vi "Acq Configure Pretrigger Period.vi"(0 "session in":refnum<class "Digitizer Control.lvclass">, 1 "desired pre-trigger period (s)":dbl, 2 "TClk period (s)":dbl, 5 "error in (no error)":errorcluster) -> (14 "session out":refnum<class "Digitizer Control.lvclass">, 15 "actual pre-trigger period (s)":dbl, 16 "configured pre-trigger period (s)":dbl, 17 "additional samples to acquire (samples)":i64, 19 "error out":errorcluster)   [LabVIEW 2021, in "Digitizer Control.lvclass"]
doc: "Configures the acquisition pre-trigger period.\n\nInputs:\n\n<B>session in</B>: The device session.\n\n<B>desired pre-trigger period (s)</B>: The desired pre-trigger period, in seconds, to acquire before recognizing the start trigger. The actual pre-trigger period is returned on the <B>actual pre-trigger period (s)</B> output.\n\n<B>TClk period (s)</B>: The TClk clock period in seconds. TClk synchronized acquisitions have an inherent trigger response latency that is between 1-2 TClk periods. The latency can be compensated by acquiring additional pre-trigger samples and keeping only latency worth of the additional pre-trigger samples. Set this input to the TClk period to compensate for the trigger latency (following the <B>niTClk Synchronize.vi</B> call, read the Actual TClk:Period propery of a tclk session passed to the <B>niTClk Synchronize.vi</B> using a Property Node and pass the returned value on this input), this will increase the pre-trigger period configured on the FPGA Target by 2*<B>TClk period (s)</B>. The FPGA Target can record the actual trigger response latency for each trigger by enabling the trigger delay tracking (using the <B>trigger delay tracking enable</B> input of the <B>Acq Configure Transfer.vi</B>). The recorded latency values can be fetched by the <B>Acq Fetch Trigger Delay.vi</B>, which also returns the number of samples to remove from the beginning of the acquired waveform to keep only <B>actual pre-trigger period (s)</B> worth of pre-trigger samples.\n\nOutputs:\n\n<B>session out</B>: The device session passed on the <B>session in</B> input.\n\n<B>actual pre-trigger period (s)</B>: The actual pre-trigger period, in seconds.\n\n<B>configured pre-trigger period (s)</B>: The pre-trigger period configured on the FPGA Target, given in seconds, including the additional pre-trigger period for the TClk trigger response latency compensation (this output equals to <B>actual pre-trigger period (s)</B> + 2 * <B>TClk period (s)</B>).\n\n<B>additional samples to acquire (samples)</B>: The number of additional samples to acquire for the TClk trigger response latency compensation. This output is valid only if the <B>Acq Configure Channel.vi</B> has been already called on the session, otherwise this output returns zero."
uses:
  Digitizer Control.lvclass
  Digitizer Control.lvclass/Digitizer Control.ctl
  <vilib>/Utility/error.llb/Error Cluster From Error Code.vi
  <vilib>/rvi/errors/niLvFpgaAdjustHostInterfaceError.vi
  <vilib>/rvi/interface/nirviReadWriteControl/nirviReadWriteControl.xnode
  <vilib>/ErrorRing/Error Ring.xnode
  NiFpgaLv.dll
  <vilib>/rvi/interface/Simulation/niFpgaSimulationCallBeginRW.vi
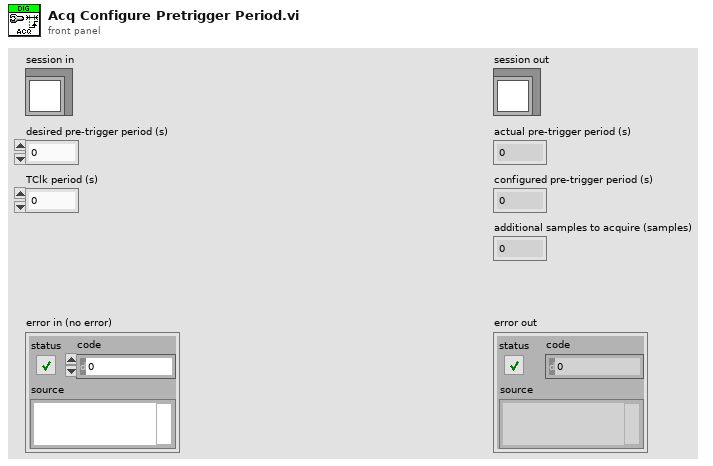
[diagram p1: front panel]
types:
  T1 = typedef "Digitizer Control.lvclass/Acq Session Data.ctl" = cluster{"ADC sampling rate":dbl, "SCTL rate":dbl, "DMA element size (bits)":i32, "sample size (bits)":i32[], "DMA/memory interface width (DMA elements)":i32, "transfer size (bits)":i32[], "stream instance":i32[], "trigger instance":u32, "group delay (s)":dbl, "data delay (s)":dbl, "target delay (s)":dbl, "trigger tracking enabled":bool, "channel configured":bool, "enabled channels":bool[], "transfer configured":bool, "dsp bypass":bool, "fractional decimator input rate":dbl, "fractional decimator output rate":dbl, "sample scale factor":dbl[], "memory size":u64[], "FIFO size":u64}
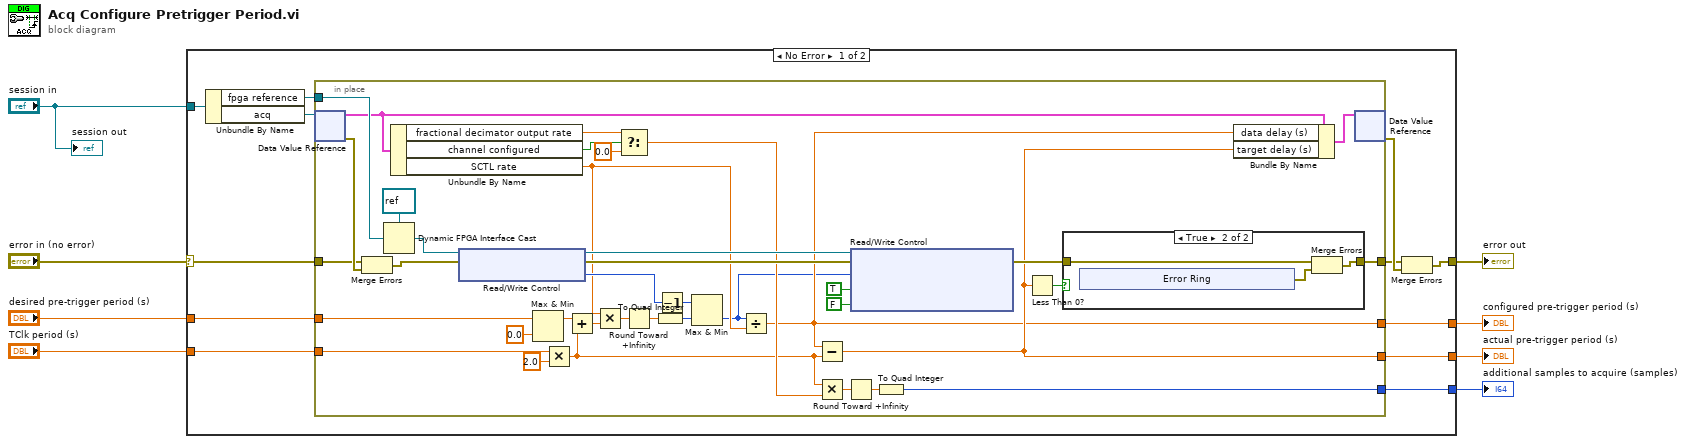
[diagram p0: block diagram]
diagram:
  n1 = case shown="No Error" "error in (no error)" {
    selector: "error in (no error)" -> [w16 w68]
    tunnel: [w10 w68] -> w7
    tunnel: "session in" -> [w19 _]
    tunnel: "TClk period (s)" -> [w14 _]
    tunnel: "desired pre-trigger period (s)" -> [w13 _]
    tunnel: [w12 _] -> w3
    tunnel: [w11 _] -> w2
    tunnel: [w9 _] -> w1
    frame No Error {
      n2 = Unbundle By Name(w19) -> ("fpga reference"=w18:refnum<k20>, "acq"=w17:refnum<data-value>)
      n3 = in-place {
        in-place-border: w18 -> [w52]
        in-place-border: w16 -> [w54]
        in-place-border: [w34] -> w15
        in-place-border: w14 -> [w48]
        in-place-border: w13 -> [w38]
        in-place-border: [w28] -> w12
        in-place-border: [w33] -> w11
        in-place-border: [w25] -> w9
        n4 = in-place-dvr #1(w17) -> (w40:T1, w55:errorcluster)
        n5 = Merge Errors(w54, w55) -> (w53:errorcluster)
        n6 = Dynamic FPGA Interface Cast(Session In=refnum<k20> refnum ("Type"), Type=w52) -> (Session Out=w51:refnum<k20>)
        n7 = Unbundle By Name(w40) -> ("fractional decimator output rate"=w31:dbl, "channel configured"=w32:bool, "SCTL rate"=w41:dbl)
        n8 = xnode "Read/Write Control"("FPGA VI Reference In"=w51, "error in"=w53) -> ("FPGA VI Reference Out"=w56:refnum<k20>, "error out"=w57:errorcluster, "acq.maximum delay"=w49:u16)
        n9 = Max & Min(x=w38, y=0.0) -> (max(x,y)=w37:dbl)  [unwired: 1 out]
        n10 = Multiply(x=w48, y=2.0 ("x")) -> (x*y=w21:dbl)
        n11 = Add(x=w37, y=w21) -> (x+y=w45:dbl)
        n12 = Multiply(x=w41, y=w45) -> (x*y=w44:dbl)
        n13 = Select(t=w31, s=w32, f=0.0) -> (s? t:f=w30:dbl)
        n14 = Round Toward +Infinity(x=w44) -> (ceil(x): smallest int >= x=w43:dbl)
        n15 = To Quad Integer(1:w43) -> (0:w42:i64)
        n16 = Decrement(x=w49) -> (x-1=w46:u16)
        n17 = Max & Min(x=w46, y=w42) -> (min(x,y)=w24:i64)  [unwired: 1 out]
        n18 = Divide(x=w24, y=w41) -> (x/y=w28:dbl)
        n19 = Subtract(x=w28, y=w21) -> (x-y=w33:dbl)
        n20 = Multiply(x=w21, y=w30) -> (x*y=w27:dbl)
        n21 = Round Toward +Infinity(x=w27) -> (ceil(x): smallest int >= x=w26:dbl)
        n22 = xnode "Read/Write Control"("FPGA VI Reference In"=w56, "error in"=w57, "flexrio.buffer.delay.clocks 0"=w24, "flexrio.buffer.delay.reset 0"=TRUE, "flexrio.buffer.delay.reset 0"=FALSE) -> ("error out"=w58:errorcluster)  [unwired: 1 out]
        n23 = To Quad Integer(1:w26) -> (0:w25:i64)
        n24 = Less Than 0?(x=w33) -> (x < 0?=w35:bool)
        n25 = case shown="True" w35 {
          tunnel: w58 -> [w59 w62]
          tunnel: [w59 w60] -> w34
          frame False {
          }
          frame True {
            n26 = xnode "Error Ring"() -> ("error out"=w61:errorcluster)
            n27 = Merge Errors(w62, w61) -> (w60:errorcluster)
          }
        }
        n28 = Bundle By Name(cluster=w40, "data delay (s)"=w28, "target delay (s)"=w33) -> (w39:T1)
        n29 = in-place-dvr #1(w39) -> (w20:errorcluster)  [unwired: 1 out]
      }
      n30 = Merge Errors(w15, w20) -> (w10:errorcluster)
    }
    frame Error {
    }
  }
  "error out" <- w7
  "actual pre-trigger period (s)" <- w2
  "configured pre-trigger period (s)" <- w3
  "additional samples to acquire (samples)" <- w1
  "session out" <- "session in"
